vi "Agilent Extract Station Data.vi"() -> ()   [LabVIEW 2009]
panel:
  out "Data":dbl[](array[numeric])
  in  "Com Port, Station":i32
  in  "Agilent Station Data Index Array":i32[][](array[numeric])
  in  "Current Agilent Data":dbl[](array[numeric])
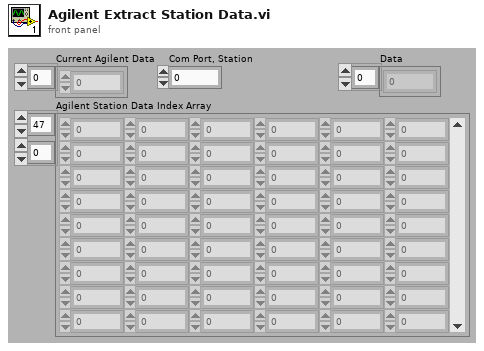
[diagram p1: front panel]
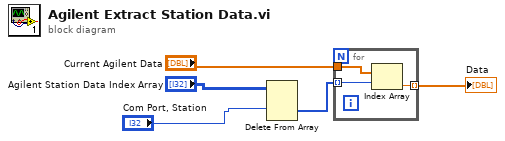
[diagram p0: block diagram]
diagram:
  n1 = Delete From Array(array="Agilent Station Data Index Array", index (row)="Com Port, Station") -> (deleted portion=w4:i32[])  [unwired: 2 in, 1 out]
  n2 = for {
    tunnel: "Current Agilent Data" -> [w8]
    tunnel: w4 -> [w7] mode=indexing
    tunnel: [w6] -> w5 mode=indexing
    n3 = Index Array(array=w8, index=w7) -> (element=w6:dbl)
  }
  "Data" <- w5
